vi "Convert To MicroVolts.vi"(8 "error in (no error)":errorcluster, 10 "Raw Data":i32[](array[numeric]), 11 "DataReceiver in":refnum<class "DataReceiver.lvclass">) -> (0 "error out":errorcluster, 2 "microVolts":dbl[](array[numeric]), 3 "DataReceiver out":refnum<class "DataReceiver.lvclass">)   [LabVIEW 2010, in "DataReceiver.lvclass"]
uses:
  DataReceiver.lvclass
  DataReceiver.lvclass/DataReceiver.ctl
  <vilib>/Analysis/polynomials.llb/1D Polynomial Evaluation (DBL).vi
  <vilib>/Analysis/NI_AALPro.lvlib
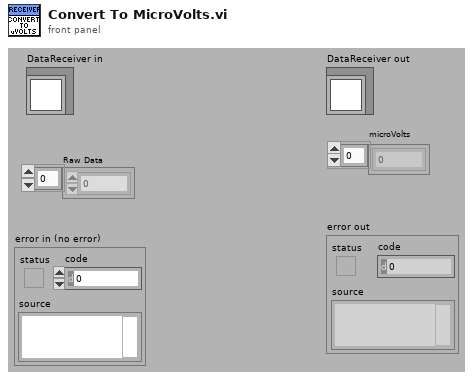
[diagram p1: front panel]
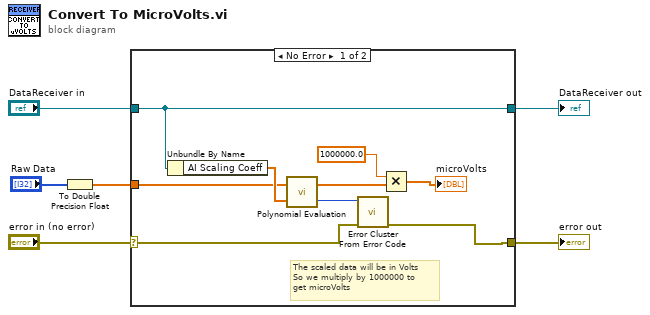
[diagram p0: block diagram]
diagram:
  n1 = To Double Precision Float(number="Raw Data") -> (double precision float=w1:dbl[])
  n2 = case shown="No Error" "error in (no error)" {
    selector: "error in (no error)" -> [w11 w17]
    tunnel: [w10 w17] -> w5
    tunnel: [w15 w16] -> w3
    tunnel: "DataReceiver in" -> [w15 w16]
    tunnel: w1 -> [w13 _]
    frame No Error {
      # "The scaled data will be in Volts\nSo we multiply by 1000000 to \nget microVolts"
      n3 = Unbundle By Name(w15) -> ("AI Scaling Coeff"=w14:dbl[])
      n4 = call-poly <vilib>:"Polynomial Evaluation.vi"("P(x)"=w14, "A"=w13) -> ("error"=w12:i32, "P(A)"=w9:dbl[])
      n5 = call <vilib>:"Error Cluster From Error Code.vi"("error in (no error)"=w11, "error code (0)"=w12) -> ("error out"=w10:errorcluster)  [unwired: 7 in]
      n6 = Multiply(x=1000000.0, y=w9) -> (x*y=→"microVolts":dbl[])
    }
    frame Error {
    }
  }
  "error out" <- w5
  "DataReceiver out" <- w3
